vi "createPlotString.vi"(9 "current plot number":i32, 10 "Plot Data":T1, 11 "plot string in":string) -> (3 "plot string out":string)   [LabVIEW 2012]
uses:
  pgfPlotPlot_tdef.ctl
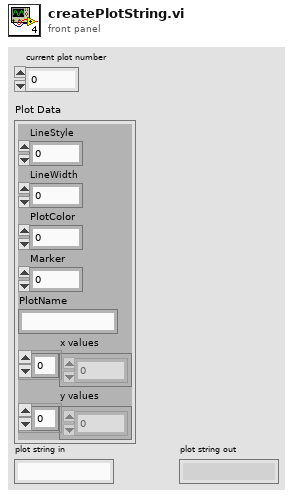
[diagram p1: front panel]
types:
  T1 = typedef "pgfPlotPlot_tdef.ctl" = cluster{"LineStyle":u8, "LineWidth":u8, "PlotColor":u32, "Marker":u8, "PlotName":string, "x values":dbl[], "y values":dbl[]}
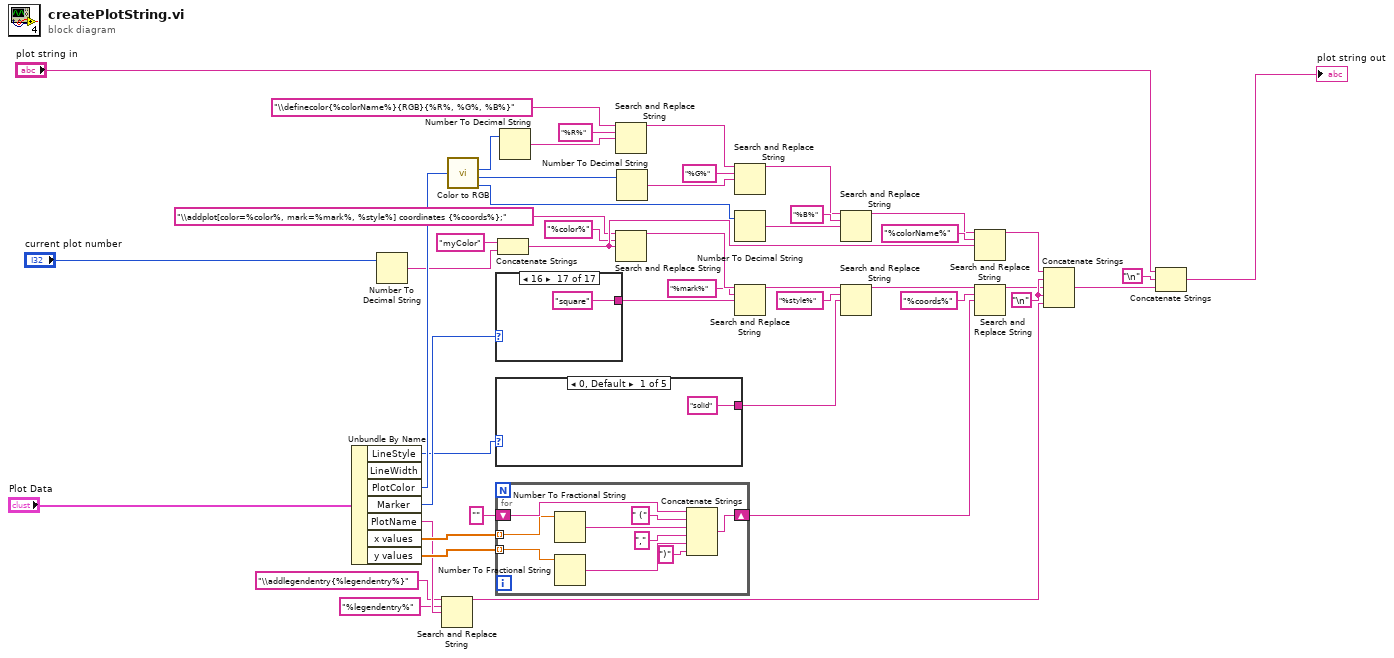
[diagram p0: block diagram]
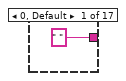
[diagram p2: hidden frame]
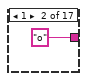
[diagram p3: hidden frame]
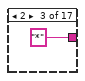
[diagram p4: hidden frame]
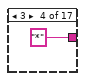
[diagram p5: hidden frame]
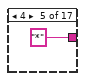
[diagram p6: hidden frame]
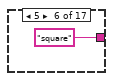
[diagram p7: hidden frame]
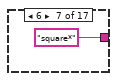
[diagram p8: hidden frame]
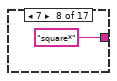
[diagram p9: hidden frame]
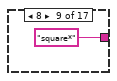
[diagram p10: hidden frame]
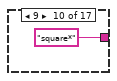
[diagram p11: hidden frame]
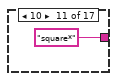
[diagram p12: hidden frame]
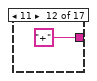
[diagram p13: hidden frame]
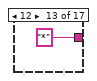
[diagram p14: hidden frame]
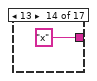
[diagram p15: hidden frame]
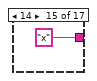
[diagram p16: hidden frame]
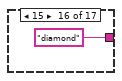
[diagram p17: hidden frame]
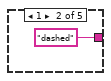
[diagram p18: hidden frame]
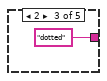
[diagram p19: hidden frame]
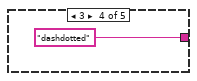
[diagram p20: hidden frame]
diagram:
  w37 = "\n"
  n1 = Unbundle By Name("Plot Data") -> ("LineStyle"=w42:u8, "PlotColor"=w43:u32, "Marker"=w44:u8, "PlotName"=w45:string, "x values"=w46:dbl[], "y values"=w47:dbl[])  [unwired: 1 out]
  n2 = Number To Decimal String(number="current plot number") -> (decimal integer string=w29:string)  [unwired: 1 in]
  n3 = Search and Replace String(input string="\\addlegendentry{%legendentry%}", search string="%legendentry%", replace string=w45) -> (result string=w40:string)  [unwired: 5 in, 3 out]
  n4 = call <vilib>:"Color to RGB.vi"("Color"=w43) -> ("R"=w19:u8, "G"=w20:u8, "B"=w21:u8)  [unwired: 1 out]
  n5 = case shown="16" w44 {
    tunnel: [" " "o" "*" "*" "*" "square" "square*" "square*" "square*" "square*" "square*" "+" "*" "x" "x" "diamond" "square"] -> w13
    frame 0, Default {
    }
    frame 1 {
    }
    frame 2 {
    }
    frame 3 {
    }
    frame 4 {
    }
    frame 5 {
    }
    frame 6 {
    }
    frame 7 {
    }
    frame 8 {
    }
    frame 9 {
    }
    frame 10 {
    }
    frame 11 {
    }
    frame 12 {
    }
    frame 13 {
    }
    frame 14 {
    }
    frame 15 {
    }
    frame 16 {
    }
  }
  n6 = case shown="0, Default" w42 {
    tunnel: ["solid" "dashed" "dotted" "dashdotted" "dashdotdotted"] -> w12
    frame 0, Default {
    }
    frame 1 {
    }
    frame 2 {
    }
    frame 3 {
    }
    frame 4 {
    }
  }
  n7 = for {
    tunnel: w47 -> [w74] mode=indexing
    tunnel: w46 -> [w75] mode=indexing
    shift-right: [w77] -> w35
    shift-left: "" -> [w78]
    n8 = Number To Fractional String(number=w75) -> (F-format string=w73:string)  [unwired: 3 in]
    n9 = Number To Fractional String(number=w74) -> (F-format string=w71:string)  [unwired: 3 in]
    n10 = Concatenate Strings(w78, " (" ("string"), w73, "," ("string"), w71, ")" ("string")) -> (w77:string)
  }
  n11 = Concatenate Strings("myColor" ("replace string (\"\")"), w29) -> (w34:string)
  n12 = Number To Decimal String(number=w19) -> (decimal integer string=w14:string)  [unwired: 1 in]
  n13 = Search and Replace String(input string="\\definecolor{%colorName%}{RGB}{%R%, %G%, %B%}", search string="%R%", replace string=w14) -> (result string=w17:string)  [unwired: 5 in, 3 out]
  n14 = Search and Replace String(input string="\\addplot[color=%color%, mark=%mark%, %style%] coordinates {%coords%};", search string="%color%", replace string=w34) -> (result string=w6:string)  [unwired: 5 in, 3 out]
  n15 = Number To Decimal String(number=w20) -> (decimal integer string=w15:string)  [unwired: 1 in]
  n16 = Search and Replace String(input string=w17, search string="%G%", replace string=w15) -> (result string=w18:string)  [unwired: 5 in, 3 out]
  n17 = Number To Decimal String(number=w21) -> (decimal integer string=w16:string)  [unwired: 1 in]
  n18 = Search and Replace String(input string=w6, search string="%mark%", replace string=w13) -> (result string=w7:string)  [unwired: 5 in, 3 out]
  n19 = Search and Replace String(input string=w18, search string="%B%", replace string=w16) -> (result string=w22:string)  [unwired: 5 in, 3 out]
  n20 = Search and Replace String(input string=w7, search string="%style%", replace string=w12) -> (result string=w8:string)  [unwired: 5 in, 3 out]
  n21 = Search and Replace String(input string=w22, search string="%colorName%", replace string=w34) -> (result string=w30:string)  [unwired: 5 in, 3 out]
  n22 = Search and Replace String(input string=w8, search string="%coords%", replace string=w35) -> (result string=w31:string)  [unwired: 5 in, 3 out]
  n23 = Concatenate Strings(w30, w37, w31, w37, w40) -> (w32:string)
  n24 = Concatenate Strings("plot string in", "\n", w32) -> (→"plot string out":string)
